vi "Append to Header and Fooder [ ].vi"(0 "PDF Report IN":refnum<class "PDF Report Class.lvclass">, 5 "Header and Footer":T1={"Header or Footer"=enum."Header", "Start page"=1, "Start with #"=0, "Type"=enum."Text", "Alignment"=enum."Center", "Vertical Alignement"=enum."BOTTOM", "Line spacing"=enum."2.0", "Image (%)"=100.0, "Page #"={"Text 1"="", "Text 2"="", "Text 3"=""}, "Text"="", "Path"="", "Font"={"Name"="Helvetica", "Size"=12.0, "Color"=0, "Style"={"Bold"=FALSE, "Italic"=FALSE, "Underline"=FALSE, "Strikeout"=FALSE}, "Type"={"Type&direction"=enum."Select", "Embedded"=FALSE, "Encoding"=""}}, "Font refnum"=refnum, "Line"={"Line"=enum."No line", "Thickness (points)"=0.0, "Colour"=0}, "Vert margin"=14.173, "Hyperlink"=""}, 11 "error in (no error)":errorcluster) -> (4 "PDF Report OUT":refnum<class "PDF Report Class.lvclass">, 15 "error out":errorcluster)   [LabVIEW 2019, in "Exaprom PDF.lvlib"]
doc: "Version 1.1\nDeveloped by Jean-Marc Simard\nCopyright © 2012, Exaprom Inc.\nAll rights reserved.\nLicense: BSD\n\nWith iTextSharp 4.1.6 (http://itextsharp.sourceforge.net)\nunder Mozilla Public License Version 1.1\n(http://www.mozilla.org/MPL/MPL-1.1.html)"
uses:
  Exaprom PDF.lvlib
  LV Class/PDF Report Class/PDF Report Class.lvclass
  LV Class/Header and Footer Class/VIs/Controls/Header Footer cluster V2.ctl
  Controls/Header, Footer and Watermark Controls/Header or Footer.ctl
  Controls/Header, Footer and Watermark Controls/Header Footer Type.ctl
  Controls/Header, Footer and Watermark Controls/Header footer horiz alignment.ctl
  Controls/Table Controls/Cell Vertical alignment.ctl
  Controls/Text Controls/Line spacing.ctl
  Controls/Header, Footer and Watermark Controls/Page number.ctl
  Controls/Font Controls/Font complete cluster horizontal.ctl
  Controls/Font Controls/Font size.ctl
  Controls/Font Controls/Font color.ctl
  Controls/Font Controls/Type and encoding.ctl
  Controls/Text Controls/Unicode/Type and run direction.ctl
  C:/work/niobrara_lv/labview pdf writer fixing/DLL/itextsharp.dll
  DLL/itextsharp.dll
  Controls/Header, Footer and Watermark Controls/Header Footer Line.ctl
  LV Class/Header and Footer Class/Header and Footer Class.lvclass
panel:
  # "X"
  # "Y"
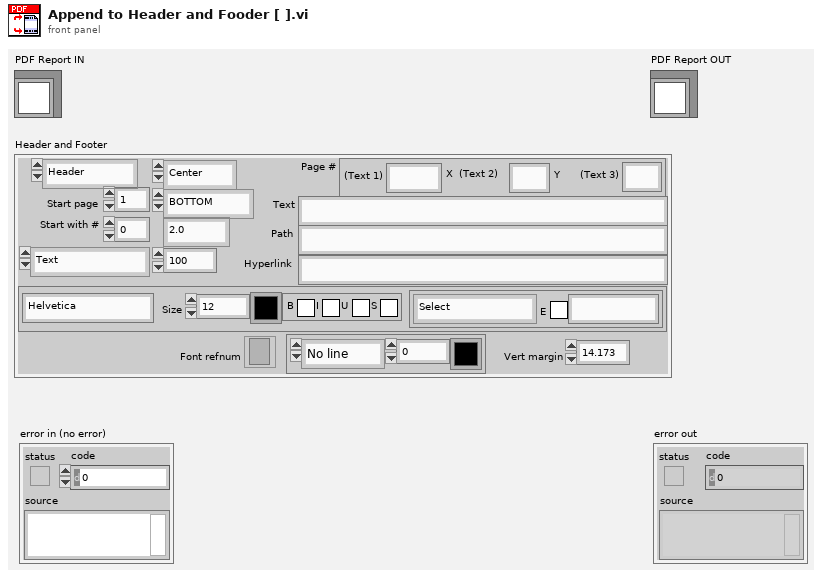
[diagram p1: front panel]
types:
  T1 = typedef "Exaprom PDF.lvlib/Header and Footer Class.lvclass/Header Footer cluster V2.ctl" = cluster{"Header or Footer":T2, "Start page":i32, "Start with #":i32, "Type":T3, "Alignment":T4, "Vertical Alignement":T5, "Line spacing":T6, "Image (%)":sgl, "Page #":T7, "Text":string, "Path":string, "Font":T8, "Font refnum":refnum<k24>, "Line":cluster{"Line":T13, "Thickness (points)":sgl, "Colour":T10}, "Vert margin":dbl, "Hyperlink":string}
  T2 = typedef "Exaprom PDF.lvlib/Header or Footer.ctl" = enum16{"Header", "Footer"}
  T3 = typedef "Exaprom PDF.lvlib/Header Footer Type.ctl" = enum16{"Select", "Text", "Text + hyperlink", "Page number", "Image", "Image + hyperlink"}
  T4 = typedef "Exaprom PDF.lvlib/Header footer horiz alignment.ctl" = enum16{"Left", "Center", "Right"}
  T5 = typedef "Exaprom PDF.lvlib/Cell Vertical alignment.ctl" = enum16{"TOP", "MIDDLE", "BOTTOM"}
  T6 = typedef "Exaprom PDF.lvlib/Line spacing.ctl" = enum16{"Select", "1.0", "1.5", "2.0"}
  T7 = typedef "Exaprom PDF.lvlib/Page number.ctl" = cluster{"Text 1":string, "Text 2":string, "Text 3":string}
  T8 = typedef "Exaprom PDF.lvlib/Font complete cluster horizontal.ctl" = cluster{"Name":string, "Size":T9, "Color":T10, "Style":cluster{"Bold":bool, "Italic":bool, "Underline":bool, "Strikeout":bool}, "Type":T11}
  T9 = typedef "Exaprom PDF.lvlib/Font size.ctl" = sgl
  T10 = typedef "Exaprom PDF.lvlib/Font color.ctl" = u32
  T11 = typedef "Exaprom PDF.lvlib/Type and encoding.ctl" = cluster{"Type&direction":T12, "Embedded":bool, "Encoding":string}
  T12 = typedef "Exaprom PDF.lvlib/Type and run direction.ctl" = enum16{"Select", "ASCII", "UTF-16", "UTF-16 (default)", "UTF-16 (LTR)", "UTF-16 (RTL)"}
  T13 = typedef "Exaprom PDF.lvlib/Header Footer Line.ctl" = enum16{"No line", "Horizontal line"}
  T14 = typedef "Exaprom PDF.lvlib/Header and Footer Class.lvclass/Header Footer [ ] V2.ctl" = T1[]
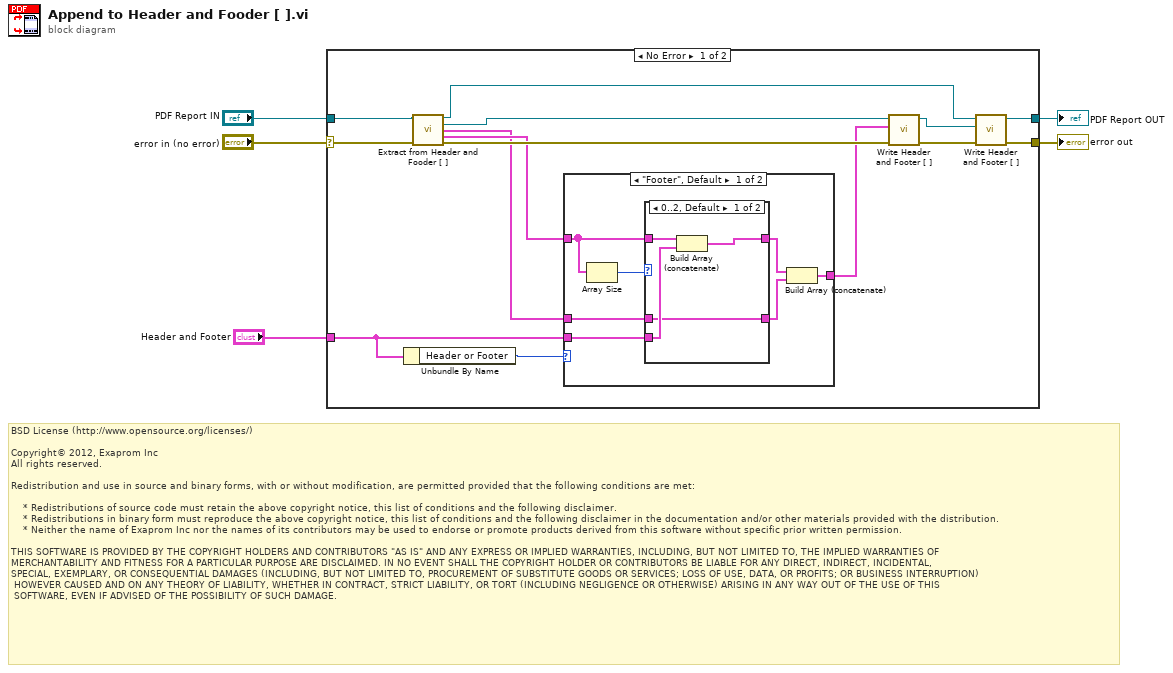
[diagram p0: block diagram]
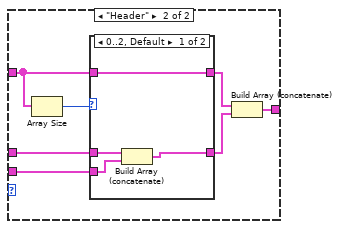
[diagram p3: hidden frame]
diagram:
  # "BSD License (http://www.opensource.org/licenses/)\n\nCopyright© 2012, Exaprom Inc\nAll rights reserved.\n\nRedistribution and use in source and binary forms, with or without modification, are permitted provided that the following conditions are met:\n\n    * Redistributions of source code must retain the above copyright notice, this list of conditions and the following disclaimer.\n    * Redistributions in binary form must reproduce the above copyright notice, this list of conditions and the following disclaimer in the documentation and/or other materials provided with the distribution.\n    * Neither the name of Exaprom Inc nor the names of its contributors may be used to endorse or promote products derived from this software without specific prior written permission.\n\nTHIS SOFTWARE IS PROVIDED BY THE COPYRIGHT HOLDERS AND CONTRIBUTORS \"AS IS\" AND ANY EXPRESS OR IMPLIED WARRANTIES, INCLUDING, BUT NOT LIMITED TO, THE IMPLIED WARRANTIES OF \nMERCHANTABILITY AND FITNESS FOR A PARTICULAR PURPOSE ARE DISCLAIMED. IN NO EVENT SHALL THE COPYRIGHT HOLDER OR CONTRIBUTORS BE LIABLE FOR ANY DIRECT, INDIRECT, INCIDENTAL,\nSPECIAL, EXEMPLARY, OR CONSEQUENTIAL DAMAGES (INCLUDING, BUT NOT LIMITED TO, PROCUREMENT OF SUBSTITUTE GOODS OR SERVICES; LOSS OF USE, DATA, OR PROFITS; OR BUSINESS INTERRUPTION)\n HOWEVER CAUSED AND ON ANY THEORY OF LIABILITY, WHETHER IN CONTRACT, STRICT LIABILITY, OR TORT (INCLUDING NEGLIGENCE OR OTHERWISE) ARISING IN ANY WAY OUT OF THE USE OF THIS\n SOFTWARE, EVEN IF ADVISED OF THE POSSIBILITY OF SUCH DAMAGE."
  n1 = case shown="No Error" "error in (no error)" {
    selector: "error in (no error)" -> [w10 w47]
    tunnel: "PDF Report IN" -> [w9 w46]
    tunnel: [w15 w46] -> w4
    tunnel: [w14 w47] -> w3
    tunnel: "Header and Footer" -> [w12 _]
    frame No Error {
      n2 = Unbundle By Name(w12) -> ("Header or Footer"=w13:T2)
      n3 = call "Extract from Header and Fooder [ ].vi"("PDF Report IN"=w9, "error in (no error)"=w10) -> ("PDF Report OUT"=w8:refnum<class "PDF Report Class.lvclass">, "Header and Footer duplicate"=w16:refnum<class "Header and Footer Class.lvclass">, "Header [ ]"=w6:T14, "Footer [ ]"=w7:T14, "error out"=w19:errorcluster)  [unwired: 9 in]
      n4 = case shown="\"Footer\", Default" w13 {
        tunnel: w7 -> [w25 w38]
        tunnel: w6 -> [w24 w37]
        tunnel: w12 -> [w23 w36]
        tunnel: [w20 w33] -> w11
        frame "Footer", Default {
          n5 = Array Size(array=w25) -> (size(s)=w26:i32)
          n6 = case shown="0..2, Default" w26 {
            tunnel: w25 -> [w30 w32]
            tunnel: w24 -> [w28 w31]
            tunnel: w23 -> [w29 _]
            tunnel: [w28 w31] -> w21
            tunnel: [w27 w32] -> w22
            frame 0..2, Default {
              n7 = Build Array (concatenate)(w30, w29) -> (w27:T14)
            }
            frame 3.. {
            }
          }
          n8 = Build Array (concatenate)(w22, w21) -> (w20:T14)
        }
        frame "Header" {
          n9 = Array Size(array=w38) -> (size(s)=w39:i32)
          n10 = case shown="0..2, Default" w39 {
            tunnel: w38 -> [w40 w45]
            tunnel: w37 -> [w43 w44]
            tunnel: w36 -> [w42 _]
            tunnel: [w41 w44] -> w34
            tunnel: [w40 w45] -> w35
            frame 0..2, Default {
              n11 = Build Array (concatenate)(w43, w42) -> (w41:T14)
            }
            frame 3.. {
            }
          }
          n12 = Build Array (concatenate)(w35, w34) -> (w33:T14)
        }
      }
      n13 = call-dynamic "Write Header and Footer [ ].vi"("error in (no error)"=w19, "Header and Footer [ ]"=w11, "Header and Footer Class in"=w16) -> ("error out"=w18:errorcluster, "Header and Footer Class out"=w17:refnum<class "Header and Footer Class.lvclass">)  [unwired: 7 in]
      n14 = call-dynamic "Write Header and Footer [ ].vi"("error in (no error)"=w18, "Header and Footer Class.lvclass"=w17, "PDF Report Class in"=w8) -> ("error out"=w14:errorcluster, "PDF Report Class out"=w15:refnum<class "PDF Report Class.lvclass">)  [unwired: 7 in]
    }
    frame Error {
    }
  }
  "PDF Report OUT" <- w4
  "error out" <- w3
